vi "ReadOutputMatrixFIFO.vi"(8 "Matrix length (in)":i32, 11 "Memory In":refnum<k21>="OutputMatrix1") -> ()   [LabVIEW 2012]
uses:
  <vilib>/rvi/interface/RandomDataEmulation/nirviRandomDataFPGAFIFO.vi
  <vilib>/rvi/interface/RandomDataEmulation/niFpgaRandomDataHandleErrors.vi
  <vilib>/rvi/DataTransferAndStorage/Container/Common/niFpgaContainerExecOnDevCompGetState.vi
  <vilib>/rvi/DataTransferAndStorage/Container/Common/niFpgaContainerGetUniqueNameForEmu.vi
  <vilib>/rvi/Memory/Memory_Emulation/niFpgaMemoryEmulationCacheClearOnFirstRun.vi
  <vilib>/rvi/Memory/Memory_Emulation/nirvimemoryEmulationManagerCache_MakeExclusive.vi
  <vilib>/rvi/Memory/Memory_Emulation/niFpgaMemoryEmulationValidateCache.vi
  <vilib>/rvi/Memory/Memory_Emulation/nirvimemoryEmulationManagerCache_ReleaseExclusive.vi
  <vilib>/rvi/Memory/Memory_Emulation/nirvimemoryEmulationManagerCache_InsertValue.vi
  <vilib>/Utility/error.llb/Clear Errors.vi
  <vilib>/rvi/Emulation/niFpgaSctlEmulationGetInTimedLoop.vi
  <vilib>/rvi/Memory/Memory_Emulation/nirvimemoryEmulationManagerCache_GetValue.vi
  <vilib>/rvi/Memory/Memory_Emulation/nirvimemoryEmulationManagerCache_SetValue.vi
  <vilib>/rvi/Emulation/niFpgaSctlEmulationResourceMgr.vi
  <vilib>/rvi/DataTransferAndStorage/Container/XNode/niFpgaContainer.xnode
  <vilib>/rvi/interface/RandomDataEmulation/nirviRandomDataFpgaReadWriteTemplate.vi
  <vilib>/rvi/Memory/Memory_Emulation/niFpgaMemoryEmulationRefIn.vi
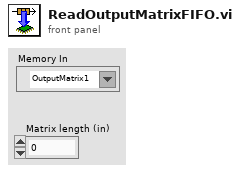
[diagram p1: front panel]
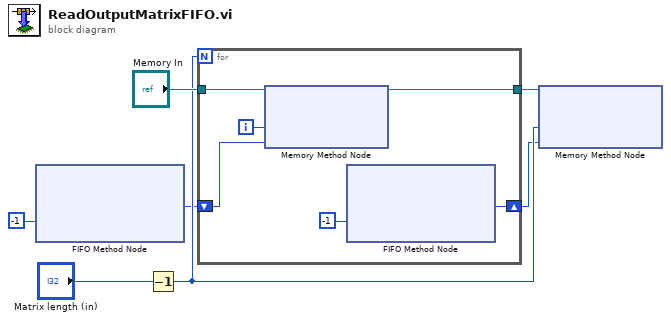
[diagram p0: block diagram]
diagram:
  n1 = xnode ("FIFO Method Node")("Timeout"=-1) -> ("Element"=w1:i16)  [unwired: 1 in, 2 out]
  n2 = Decrement(x="Matrix length (in)") -> (x-1=w5:i32)
  n3 = for {
    N: w5 -> [_]
    shift-right: [w12] -> w2
    shift-left: w1 -> [w13]
    tunnel: "Memory In" -> [w10]
    tunnel: [w9] -> w7
    i -> [w11]
    n4 = xnode ("Memory Method Node")("Address"=w11, "Data"=w13, "Memory In"=w10) -> ("Memory Out"=w9:refnum<k21>)
    n5 = xnode ("FIFO Method Node")("Timeout"=-1) -> ("Element"=w12:i16)  [unwired: 1 in, 2 out]
  }
  n6 = xnode ("Memory Method Node")("Address"=w5, "Data"=w2, "Memory In"=w7) -> ()  [unwired: 1 out]
